vi "Create.vi"(8 "error in (no error)":errorcluster) -> (0 "error out":errorcluster, 3 "Message Template out":refnum<class "Message Template.lvclass">)   [LabVIEW 2020, in "Message Template.lvclass"]
uses:
  Message Template.lvclass
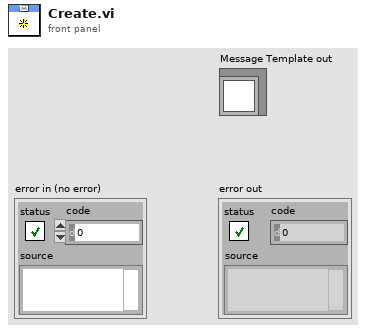
[diagram p1: front panel]
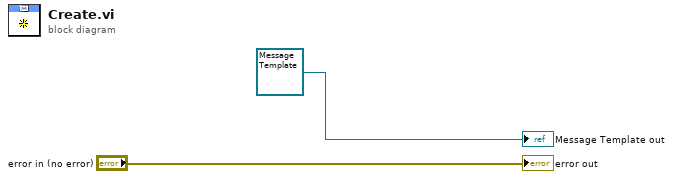
[diagram p0: block diagram]
diagram:
  "error out" <- "error in (no error)"
  "Message Template out" <- refnum<class "Message Template.lvclass"> refnum ("Message Template in")
